vi "writeLUT.vi"(9 "text":string, 11 "base path":path) -> ()   [LabVIEW 2020]
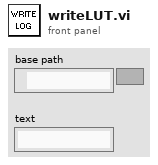
[diagram p1: front panel]
types:
  T1 = enum16{"open", "replace", "create", "open or create", "replace or create", "replace or create with confirmation"}
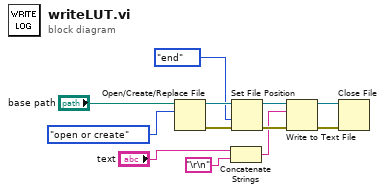
[diagram p0: block diagram]
diagram:
  n1 = Open/Create/Replace File(file path (use dialog)="base path", operation (0:open)=T1."open or create") -> (refnum out=w9:refnum<file>, error out=w6:errorcluster)  [unwired: 4 in, 1 out]
  n2 = Concatenate Strings("text", "\r\n") -> (w3:string)
  n3 = Set File Position(refnum=w9, from (0:start)=enum16{"start", "end", "current"}."end", error in=w6) -> (refnum out=w8:refnum<file>, error out=w7:errorcluster)  [unwired: 1 in]
  n4 = Write to Text File(file (use dialog)=w8, text=w3, error in=w7) -> (refnum out=w11:refnum<file>, error out=w10:errorcluster)  [unwired: 1 in, 1 out]
  n5 = Close File(refnum=w11, error in=w10) -> ()  [unwired: 2 out]
